vi "Mixer.Write String.vi"(0 "url":string="http://169.254.128.32/datastore/", 7 "value":string, 11 "error in (no error)":errorcluster) -> (15 "error out":errorcluster)   [LabVIEW 2020]
uses:
  <vilib>/httpClient/POSTBuffer.vi
  <vilib>/httpClient/LabVIEWHTTPClient.lvlib
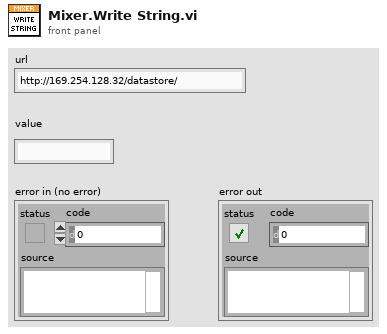
[diagram p1: front panel]
types:
  T1 = typedef "LabVIEWHTTPClient.lvlib/ClientHandle.ctl" = refnum<k1>
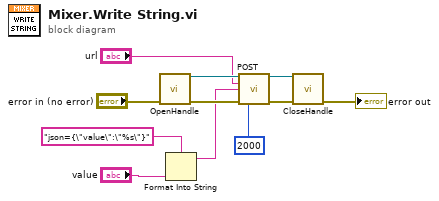
[diagram p0: block diagram]
diagram:
  n1 = call <vilib>:"OpenHandle.vi"("error in (no error)"="error in (no error)") -> ("client handle out"=w9:T1, "error out"=w8:errorcluster)  [unwired: 13 in]
  n2 = Format Into String(format string="json={\"value\":\"%s\"}" ("buffer"), "value") -> (resulting string=w4:string)  [unwired: 2 in, 1 out]
  n3 = call-poly <vilib>:"POST.vi"("client handle"=w9, "url"="url", "buffer"=w4, "error in (no error)"=w8, "timeout (10000)"=2000) -> ("client handle out"=w10:T1, "error out"=w11:errorcluster)  [unwired: 7 in, 2 out]
  n4 = call <vilib>:"CloseHandle.vi"("client handle"=w10, "error in (no error)"=w11) -> ("error out"=→"error out":errorcluster)  [unwired: 13 in]
